vi "Periodic Tasks.vi"(8 "error in":errorcluster) -> ()   [LabVIEW 2013]
doc: "This VI runs in parallel to other tasks. It can contain as many user-defined periodic loops as you need. These can carry out PID or other sorts of timed response."
uses:
  <vilib>/Rock Robotics/SystemInterfaces/Utilities/FPGA_UtilitiesLED Source.ctl
  <vilib>/Rock Robotics/SystemInterfaces/Utilities/FPGA_UtilitiesLED State.ctl
  Robot Global Data.vi
panel:
  out "Distance":dbl
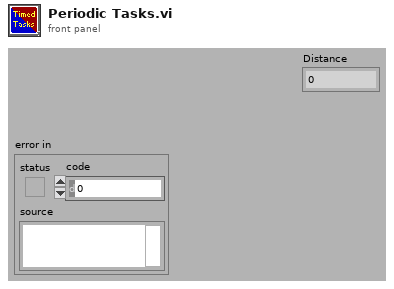
[diagram p1: front panel]
types:
  T1 = typedef "WPI_DigitalInputDevRef.ctl" = cluster{"DevStatus":errorcluster, "DIO Channel":T2, "Digital Module":T3}
  T2 = typedef "FPGA_DIOChannel.ctl" = enum8{"DIO 1", "DIO 2", "DIO 3", "DIO 4", "DIO 5", "DIO 6", "DIO 7", "DIO 8", "DIO 9", "DIO 10", "DIO 11", "DIO 12", "DIO 13", "DIO 14", "Invalid"}
  T3 = typedef "FPGA_TypedefDigitalModule.ctl" = enum16{"Digital Module 1", "Digital Module 2"}
  T4 = typedef "WPI_AnalogChannelDevRef.ctl" = cluster{"DevStatus":errorcluster, "Analog Module":T5, "Analog Channel":T6}
  T5 = typedef "FPGA_TypedefAnalogModule.ctl" = enum16{"Analog Module 1", "Analog Module 2"}
  T6 = typedef "FPGA_AIChannel.ctl" = enum8{"AI 1", "AI 2", "AI 3", "AI 4", "AI 5", "AI 6", "AI 7", "AI 8", "Invalid"}
  T7 = typedef "WPI_EncoderDevRef.ctl" = cluster{"DevStatus":errorcluster, "EncoderIndex":T8, "CounterIndex":T9, "DistancePerCount":dbl, "Decoding Type":T10}
  T8 = typedef "FPGA_EncoderIdx.ctl" = enum8{"Enc 0", "Enc 1", "Enc 2", "Enc 3", "Invalid"}
  T9 = typedef "FPGA_CounterCtrSystemIndex.ctl" = enum8{"Ctr 0", "Ctr 1", "Ctr 2", "Ctr 3", "Ctr 4", "Ctr 5", "Ctr 6", "Ctr 7", "Invalid"}
  T10 = typedef "WPI_EncoderType.ctl" = enum16{"1x", "2x", "4x"}
  T11 = typedef "FPGA_UtilitiesLED State.ctl" = enum16{"Off", "On", "Toggle"}
  T12 = typedef "FPGA_UtilitiesLED Source.ctl" = enum16{"User LED", "FPGA LED"}
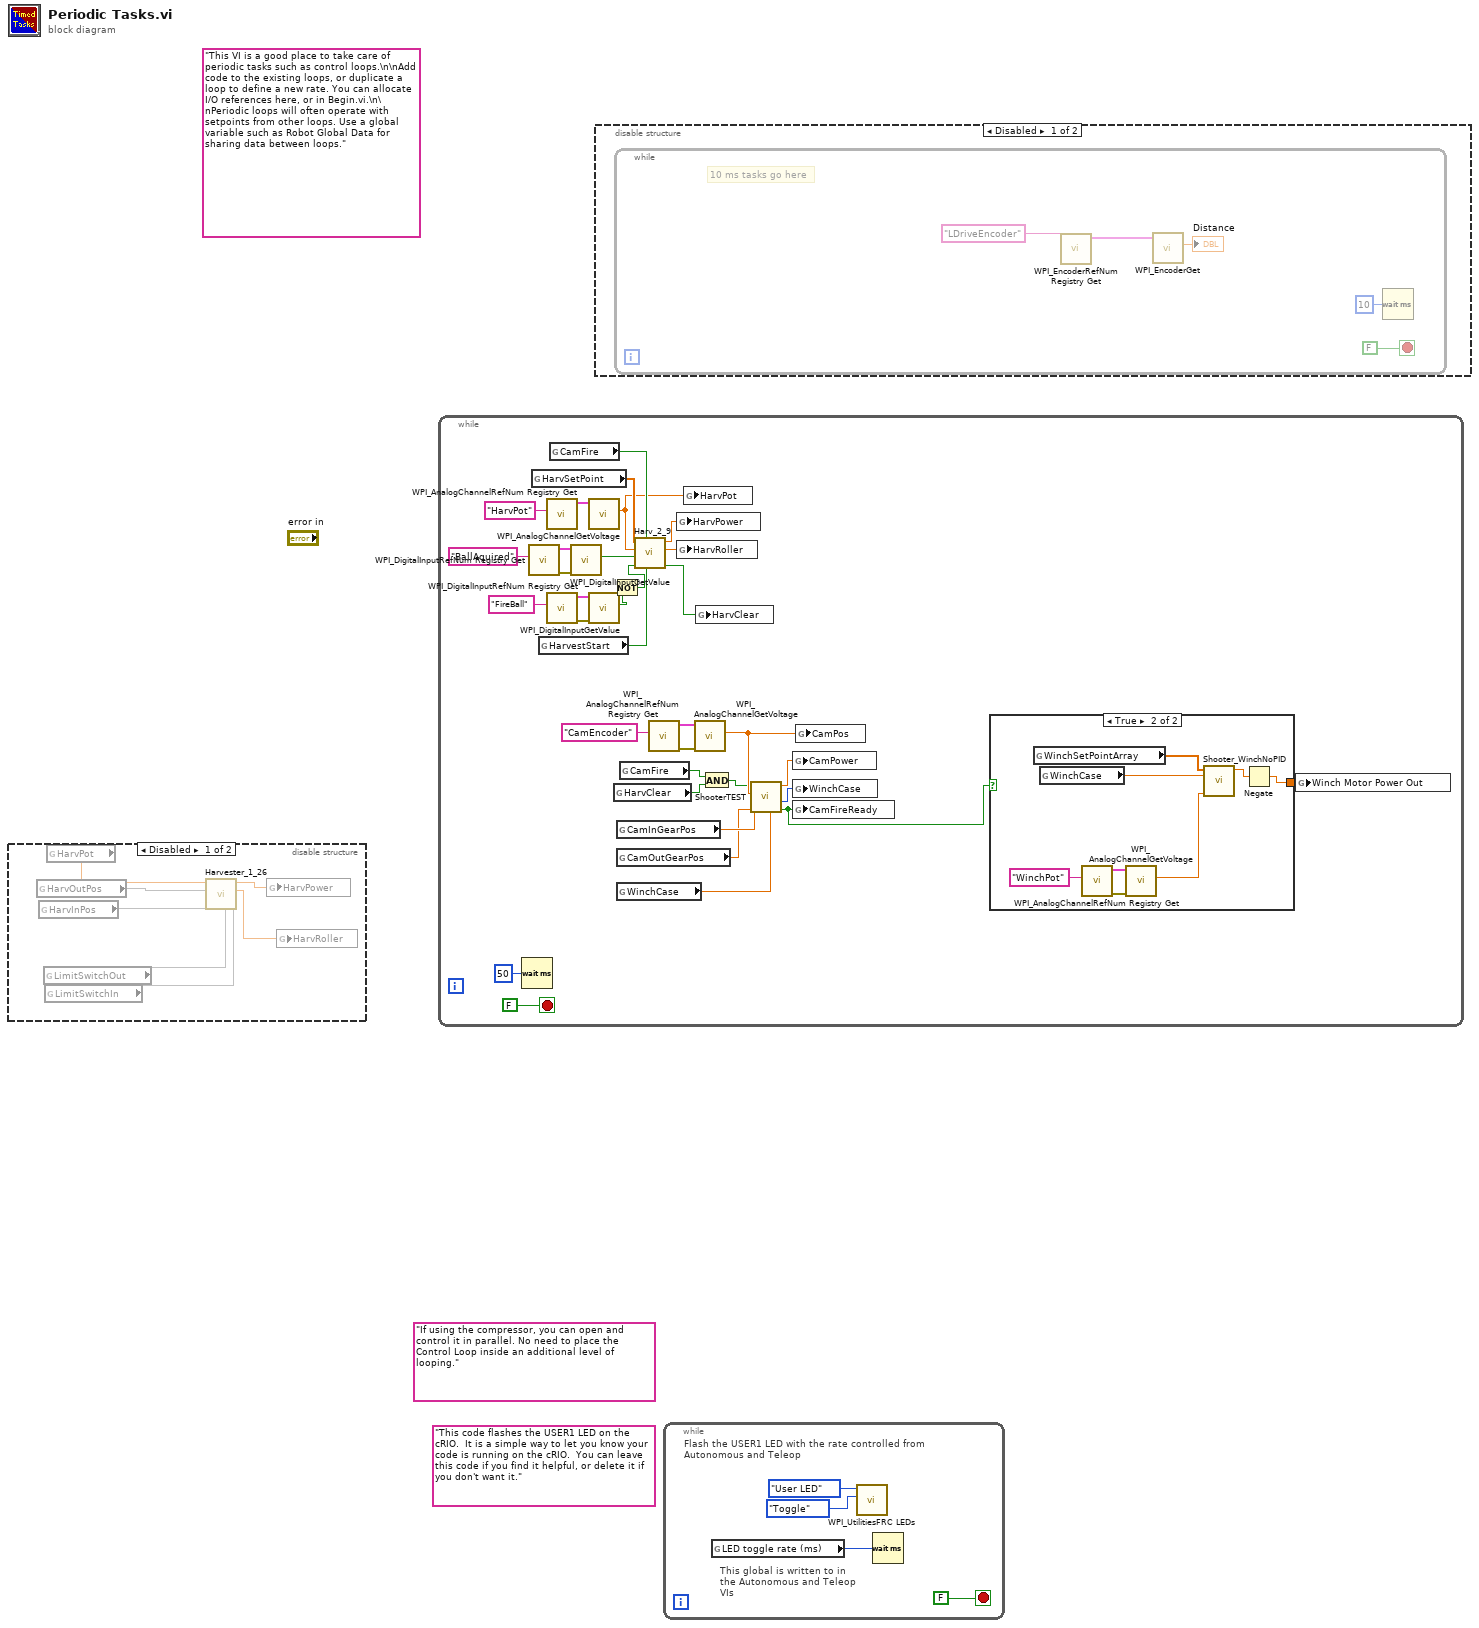
[diagram p0: block diagram]
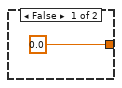
[diagram p4: hidden frame]
diagram:
  (unwired) "If using the compressor, you can open and control it in parallel. No need to place the Control Loop inside an additional level of looping."
  (unwired) "This code flashes the USER1 LED on the cRIO.  It is a simple way to let you know your code is running on the cRIO.  You can leave this code if you find it helpful, or delete it if you don't want it."
  (unwired) "This VI is a good place to take care of periodic tasks such as control loops.\n\nAdd code to the existing loops, or duplicate a loop to define a new rate. You can allocate I/O references here, or in Begin.vi.\n\nPeriodic loops will often operate with setpoints from other loops. Use a global variable such as Robot Global Data for sharing data between loops."
  n1 = disable-structure shown="Disabled" {
    frame Disabled {
      n2 = global read "Robot Global Data.vi" "HarvOutPos"() -> (w6)
      n3 = global read "Robot Global Data.vi" "HarvInPos"() -> (w5)
      n4 = global read "Robot Global Data.vi" "LimitSwitchOut"() -> (w4)
      n5 = global read "Robot Global Data.vi" "LimitSwitchIn"() -> (w3)
      n6 = global read "Robot Global Data.vi" "HarvPot"() -> (w7:dbl)
      n7 = call "Harvester_1_26.vi"("LimitSwitchIn"=w3, "LimitSwitchOut"=w4, "HarvInPos"=w5, "HarvOutPos"=w6, "HarvPot"=w7) -> ("HarvRoller"=w2:dbl, "HarvPower"=w1:dbl)  [unwired: 5 in]
      n8 = global write "Robot Global Data.vi" "HarvPower"(w1) -> ()
      n9 = global write "Robot Global Data.vi" "HarvRoller"(w2) -> ()
    }
    frame Enabled {
    }
  }
  n10 = while {
    stop <- FALSE stop-if-true
    n11 = Wait (ms)(milliseconds to wait=u32 50) -> ()  [unwired: 1 out]
    n12 = call <vilib>:"WPI_DigitalInputRefNum Registry Get.vi"("refnum name"="BallAquired") -> ("error out"=w31:errorcluster, "DigitalInputDevRef"=w30:T1)  [unwired: 9 in]
    n13 = global read "Robot Global Data.vi" "HarvSetPoint"() -> (w16:dbl[])
    n14 = global read "Robot Global Data.vi" "HarvestStart"() -> (w17:bool)
    n15 = call <vilib>:"WPI_AnalogChannelRefNum Registry Get.vi"("refnum name"="HarvPot") -> ("AIDeviceRef"=w23:T4)  [unwired: 9 in, 1 out]
    n16 = call <vilib>:"WPI_DigitalInputRefNum Registry Get.vi"("refnum name"="FireBall") -> ("error out"=w19:errorcluster, "DigitalInputDevRef"=w20:T1)  [unwired: 9 in]
    n17 = global read "Robot Global Data.vi" "CamFire"() -> (w18:bool)
    n18 = call <vilib>:"WPI_DigitalInputGetValue.vi"("error in (no error)"=w31, "DigitalInputDevRef"=w30) -> ("Value"=w8:bool)  [unwired: 7 in, 2 out]
    n19 = call <vilib>:"WPI_AnalogChannelGetVoltage.vi"("AIDeviceRef"=w23) -> ("Voltage"=w11:dbl)  [unwired: 8 in, 2 out]
    n20 = call <vilib>:"WPI_DigitalInputGetValue.vi"("error in (no error)"=w19, "DigitalInputDevRef"=w20) -> ("Value"=w9:bool)  [unwired: 7 in, 2 out]
    n21 = Not(x=w9) -> (.not. x?=w10:bool)
    n22 = global read "Robot Global Data.vi" "HarvClear"() -> (w14:bool)
    n23 = global read "Robot Global Data.vi" "CamInGearPos"() -> (w39:dbl)
    n24 = global read "Robot Global Data.vi" "CamOutGearPos"() -> (w38:dbl)
    n25 = global read "Robot Global Data.vi" "WinchCase"() -> (w26:dbl)
    n26 = global read "Robot Global Data.vi" "CamFire"() -> (w13:bool)
    n27 = call "Harv_2_9.vi"("Harvest"=w17, "Fire"=w18, "FireBallSen"=w10, "BallAcquired"=w8, "HarvPot"=w11, "HarvSetpoints"=w16) -> ("HarvCleared"=w15:bool, "HarvRoller"=w24:dbl, "HarvPower"=w25:dbl)  [unwired: 3 in]
    n28 = call <vilib>:"WPI_AnalogChannelRefNum Registry Get.vi"("refnum name"="CamEncoder") -> ("error out"=w35:errorcluster, "AIDeviceRef"=w34:T4)  [unwired: 9 in]
    n29 = global write "Robot Global Data.vi" "HarvPower"(w25) -> ()
    n30 = global write "Robot Global Data.vi" "HarvRoller"(w24) -> ()
    n31 = global write "Robot Global Data.vi" "HarvPot"(w11) -> ()
    n32 = call <vilib>:"WPI_AnalogChannelGetVoltage.vi"("error in (no error)"=w35, "AIDeviceRef"=w34) -> ("Voltage"=w33:dbl)  [unwired: 7 in, 2 out]
    n33 = global write "Robot Global Data.vi" "HarvClear"(w15) -> ()
    n34 = And(x=w13, y=w14) -> (x .and. y?=w12:bool)
    n35 = call "ShooterTEST.vi"("WinchCaseIn"=w26, "OutGearPos"=w38, "InGearPos"=w39, "Pot"=w33, "Fire"=w12) -> ("There?"=w28:bool, "WinchCase"=w27:i32, "Power"=w37:dbl)  [unwired: 4 in]
    n36 = global write "Robot Global Data.vi" "CamPower"(w37) -> ()
    n37 = global write "Robot Global Data.vi" "WinchCase"(w27) -> ()
    n38 = global write "Robot Global Data.vi" "CamFireReady"(w28) -> ()
    n39 = global write "Robot Global Data.vi" "CamPos"(w33) -> ()
    n40 = case shown="True" w28 {
      tunnel: [0.0 ("Winch Motor Power Out") w44] -> w32
      frame False {
      }
      frame True {
        n41 = global read "Robot Global Data.vi" "WinchSetPointArray"() -> (w43:dbl[])
        n42 = global read "Robot Global Data.vi" "WinchCase"() -> (w46:dbl)
        n43 = call <vilib>:"WPI_AnalogChannelRefNum Registry Get.vi"("refnum name"="WinchPot") -> ("error out"=w49:errorcluster, "AIDeviceRef"=w50:T4)  [unwired: 9 in]
        n44 = call <vilib>:"WPI_AnalogChannelGetVoltage.vi"("error in (no error)"=w49, "AIDeviceRef"=w50) -> ("Voltage"=w47:dbl)  [unwired: 7 in, 2 out]
        n45 = call "Shooter_WinchNoPID.vi"("Winch Pot Location"=w47, "selectedCase"=w46, "SetPointArray"=w43) -> ("Winch Motor Power Out"=w45:dbl)  [unwired: 8 in]
        n46 = Negate(x=w45) -> (-x=w44:dbl)
      }
    }
    n47 = global write "Robot Global Data.vi" "Winch Motor Power Out"(w32) -> ()
  }
  n48 = disable-structure shown="Disabled" {
    frame Disabled {
      n49 = while {
        stop <- FALSE stop-if-true
        # "10 ms tasks go here"
        n50 = call <vilib>:"WPI_EncoderRefNum Registry Get.vi"("refnum name"="LDriveEncoder") -> ("EncoderDevRef"=w51:T7)  [unwired: 9 in, 1 out]
        n51 = call <vilib>:"WPI_EncoderGet.vi"("EncoderDevRef"=w51) -> ("Distance"=→"Distance":dbl)  [unwired: 5 in, 5 out]
        n52 = Wait (ms)(milliseconds to wait=u32 10) -> ()  [unwired: 1 out]
      }
    }
    frame Enabled {
    }
  }
  n53 = while {
    stop <- FALSE stop-if-true
    # "This global is written to in the Autonomous and Teleop VIs"
    # "Flash the USER1 LED with the rate controlled from Autonomous and Teleop"
    n54 = global read "Robot Global Data.vi" "LED toggle rate (ms)"() -> (w56:u32)
    n55 = call <vilib>:"WPI_UtilitiesFRC LEDs.vi"("State"=FPGA_UtilitiesLED_State."Toggle", "LED Type"=FPGA_UtilitiesLED_Source."User LED") -> ()  [unwired: 1 in, 9 out]
    n56 = Wait (ms)(milliseconds to wait=w56) -> ()  [unwired: 1 out]
  }
